vi "Stop Core.vi"(10 "final error code":i32, 11 "SpectroscopyUI in":refnum<class "SpectroscopyUI.lvclass">) -> (3 "SpectroscopyUI out":refnum<class "SpectroscopyUI.lvclass">)   [LabVIEW 2023, in "SpectroscopyUI.lvlib" / "SpectroscopyUI.lvclass"]
doc: "(<B>Filename</B>: Actor Framework.lvlib:Actor.lvclass:Stop Core.vi)\n\nDefines what the actor does before it stops. Use the <B>final error code</B> input to determine whether the actor shut down in response to an error.\n\nBy default, this method passes the Stop message along to all auto-stop nested actors. A descendant class may override this method to define additional behavior, such as shutting down any processes the actor initiated in its override of the Actor Core method."
uses:
  SpectroscopyUI.lvclass
  <vilib>/ActorFramework/Actor/Actor.lvclass
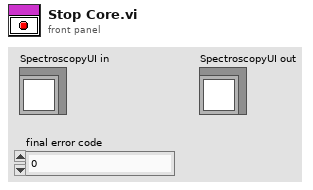
[diagram p1: front panel]
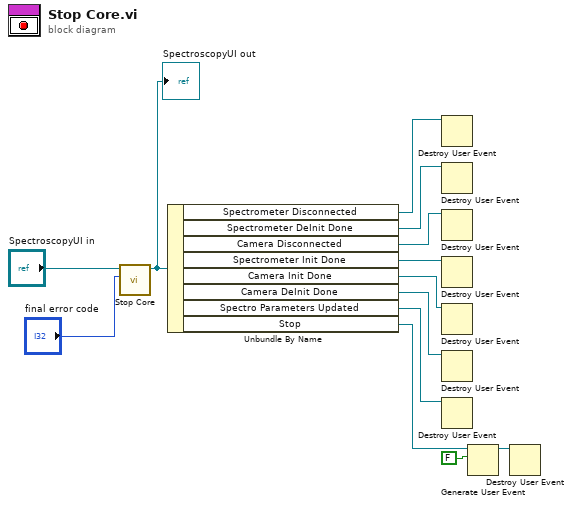
[diagram p0: block diagram]
diagram:
  n1 = call-parent "Stop Core.vi"("final error code"="final error code", "Actor in"="SpectroscopyUI in") -> ("Actor out"=w10:refnum<class "SpectroscopyUI.lvclass">)  [unwired: 9 in]
  "SpectroscopyUI out" <- w10
  n2 = Unbundle By Name(w10) -> ("Spectrometer Disconnected"=w3:refnum<user-event>, "Spectrometer DeInit Done"=w2:refnum<user-event>, "Camera Disconnected"=w1:refnum<user-event>, "Spectrometer Init Done"=w5:refnum<user-event>, "Camera Init Done"=w4:refnum<user-event>, "Camera DeInit Done"=w9:refnum<user-event>, "Spectro Parameters Updated"=w8:refnum<user-event>, "Stop"=w7:refnum<user-event>)
  n3 = Destroy User Event(user event=w3) -> ()  [unwired: 1 in, 1 out]
  n4 = Destroy User Event(user event=w2) -> ()  [unwired: 1 in, 1 out]
  n5 = Destroy User Event(user event=w1) -> ()  [unwired: 1 in, 1 out]
  n6 = Destroy User Event(user event=w5) -> ()  [unwired: 1 in, 1 out]
  n7 = Destroy User Event(user event=w4) -> ()  [unwired: 1 in, 1 out]
  n8 = Destroy User Event(user event=w9) -> ()  [unwired: 1 in, 1 out]
  n9 = Destroy User Event(user event=w8) -> ()  [unwired: 1 in, 1 out]
  n10 = Generate User Event(user event=w7, event data cluster=FALSE ("event data")) -> (user event out=w11:refnum<user-event>)  [unwired: 2 in, 1 out]
  n11 = Destroy User Event(user event=w11) -> ()  [unwired: 1 in, 1 out]
